vi "Reshape Cal Table.vi"(0 "Speaker amplitudes":dbl[](array[numeric]), 1 "Start dB SPL":dbl=60.0 format="%#_13g", 2 "End dB SPL":dbl=130.0 format="%#_13g", 5 "Frequencies":dbl[](array[numeric]), 7 "Measured dB SPL":dbl[][](array[numeric]), 11 "error in (no error)":errorcluster, 12 "dB SPL Increment":dbl=1.0 format="%#_13g") -> (4 "dB SPL Axis":dbl[](array[numeric]), 6 "Frequency Axis":dbl[](array[numeric]), 8 "Speaker amplitude":dbl[][](array[numeric]) format="%#_2p", 15 "error out":errorcluster)   [LabVIEW 2020]
doc: "Reshape Cal Table is used to convert the 3D LUT of Amplitude, Frequency and dB SPL to dB SPL along the columns and Frequency along rows where Amplitude will be the data element cell."
uses:
  <vilib>/Analysis/1siggen.llb/Ramp Pattern.vi
  <vilib>/Analysis/1siggen.llb/Ramp Pattern by Delta.vi
  <vilib>/gmath/NI_Gmath.lvlib
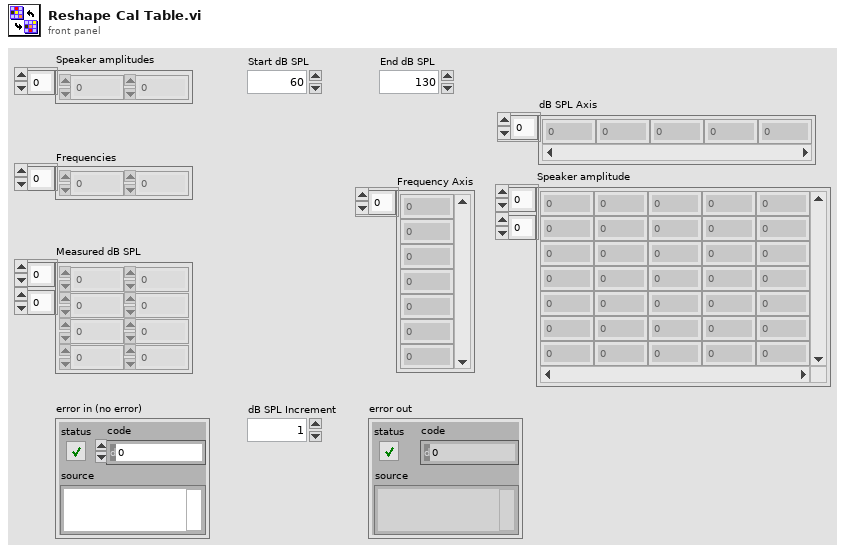
[diagram p1: front panel]
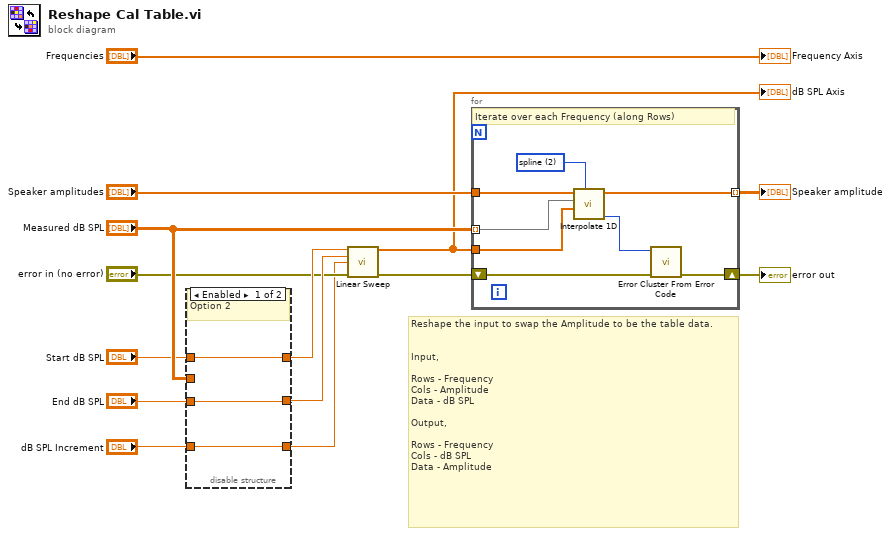
[diagram p0: block diagram]
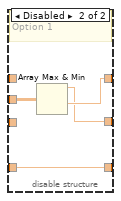
[diagram p2: hidden frame]
diagram:
  # "Reshape the input to swap the Amplitude to be the table data.\n\n\nInput,\n\nRows - Frequency\nCols - Amplitude\nData - dB SPL\n\nOutput,\n\nRows - Frequency\nCols - dB SPL\nData - Amplitude"
  n1 = disable-structure shown="Enabled" {
    disable-tunnel: "Measured dB SPL" -> [_ w21]
    disable-tunnel: [w16 w20] -> w13
    disable-tunnel: [w15 w19] -> w12
    disable-tunnel: "dB SPL Increment" -> [w17 w18]
    disable-tunnel: [w17 w18] -> w9
    disable-tunnel: "End dB SPL" -> [w15 _]
    disable-tunnel: "Start dB SPL" -> [w16 _]
    frame Enabled {
      # "Option 2"
    }
    frame Disabled {
      # "Option 1"
      n2 = Array Max & Min(array=w21) -> (max value=w19:dbl, min value=w20:dbl)  [unwired: 2 out]
    }
  }
  n3 = call "Linear Sweep.vi"("Start"=w13, "End"=w12, "Delta"=w9, "error in (no error)"="error in (no error)") -> ("Ramp Pattern"=w4:dbl[], "error out"=w8:errorcluster)  [unwired: 10 in]
  "dB SPL Axis" <- w4
  n4 = for {
    tunnel: "Measured dB SPL" -> [w25] mode=indexing
    tunnel: "Speaker amplitudes" -> [w24]
    shift-right: [w28] -> w7
    shift-left: w8 -> [w29]
    tunnel: w4 -> [w26]
    tunnel: [w23] -> w5 mode=indexing
    w22 = 2 items=["nearest", "linear", "spline", "cubic Hermite", "Lagrange"] ("method")
    # "Iterate over each Frequency (along Rows)"
    n5 = call <vilib>:"Interpolate 1D.vi"("method"=w22, "xi"=w26, "X"=w25, "Y"=w24) -> ("error"=w27:i32, "yi"=w23:dbl[])  [unwired: 5 in, 1 out]
    n6 = call <vilib>:"Error Cluster From Error Code.vi"("error in (no error)"=w29, "error code (0)"=w27) -> ("error out"=w28:errorcluster)  [unwired: 7 in]
  }
  "Speaker amplitude" <- w5
  "error out" <- w7
  "Frequency Axis" <- "Frequencies"
